vi "Main Page.vi"(8 "error in (no error)":errorcluster, 11 "Node Ptr":T2 format="%.0x") -> (0 "error out":errorcluster)   [LabVIEW 2015, in "SLSC-12201 DIO System Explorer.lvlib"]
uses:
  SLSC-12201 DIO System Explorer.lvlib
  <vilib>/NI Veristand/Custom Device API/Custom Device Item Ref.ctl
  Direction Control.ctl
  Shared/Constants.vi
  <vilib>/NI Veristand/Custom Device Tools/Custom Device Utility Library/NI VeriStand - Search for All Items by Name.vi
  <vilib>/NI Veristand/Custom Device API/Get Item Property (Boolean).vi
  <vilib>/NI Veristand/Custom Device Tools/Custom Device Utility Library/NI VeriStand - Search for Item by Name.vi
  <vilib>/NI Veristand/Custom Device API/Get Item Property (I32).vi
  <vilib>/NI Veristand/Custom Device API/Get Item Property (Variant).vi
  <vilib>/NI Veristand/Custom Device API/Set Item Property (Variant).vi
  SLSC Pinout Window.vi
  SLSC Diagram Window.vi
  <vilib>/NI Veristand/Custom Device API/Set Item Property (Boolean).vi
  <vilib>/NI Veristand/Custom Device API/Set Item Property (String).vi
  <vilib>/NI Veristand/Custom Device API/Custom Device API.lvlib
  Shared/SLSC-12201 DIO Shared.lvlib
  <vilib>/NI Veristand/Custom Device Tools/Custom Device Utility Library/Custom Device Utility Library.lvlib
panel:
  in  "Loop rate":u32
  in  "rev A":bool
  in  "SHDocVw.IWebBrowser2":refnum<k7>(container)
  out "Version":string
  in  "Direction":T1 items=["Input", "Output Source", "Output Sink", "Output Push-Pull"]
  in  "Apply":bool
  in  "Enable":bool
  in  "Disable":bool
  in  "Tab Control":enum32{"Bank 0", "Bank 1"}(tab)
  in  "Input Threshold 5V Bank 0":dbl caption="Input Threshold"
  in  "Bank0 Select Vsup":u16(ring) caption="Voltage Supply" items=["Off", "Vsup_0", "Vsup_1"]
  in  "Pullup Resistor Bank 0":bool
  in  "Input Threshold 33V Bank 0":dbl caption="Input Threshold"
  in  "Enable 5V Range Bank 0":bool
  in  "Input Threshold 5V Bank 1":dbl caption="Input Threshold"
  in  "Bank1 Select Vsup":u16(ring) caption="Voltage Supply" items=["Off", "Vsup_0", "Vsup_1"]
  in  "Enable 5V Range Bank 1":bool
  in  "Pullup Resistor Bank 1":bool
  in  "Input Threshold 33V Bank 1":dbl caption="Input Threshold"
  in  "Tree":string[](tree)
  in  "Make Static Only":bool
  in  "Title":cluster{"Section Name":string}={"Section Name"="Custom Device Properties"}
  out "Module Number":i32
  in  "Header":cluster{"Section Name":string}={"Section Name"="Custom Device Item Settings"}
  in  "Description":string
  in  "Name":string
  # "ms"
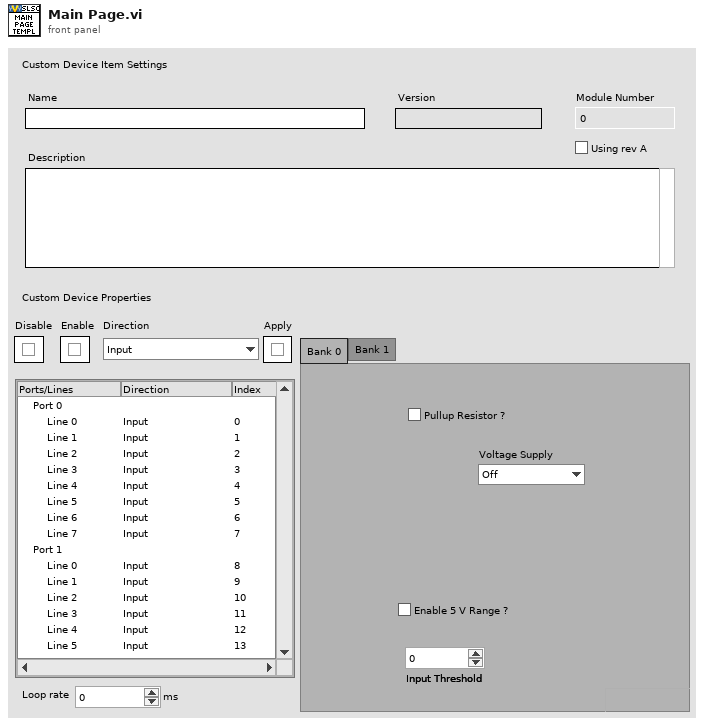
[diagram p1: front panel]
types:
  T1 = typedef "SLSC-12201 DIO System Explorer.lvlib/Direction Control.ctl" = u16
  T2 = typedef "Custom Device API.lvlib/Custom Device Item Ref.ctl" = u64
  T3 = enum8{"Enabled", "Disabled", "Disabled and Grayed Out"}
  T4 = typedef "Custom Device API.lvlib/Custom Device Channel.ctl" = cluster{"Type":T5, "Units":string, "Default Value":dbl, "Faultable":bool, "Scalable":bool}
  T5 = typedef "Custom Device API.lvlib/Custom Device Channel Type.ctl" = enum16{"Input", "Output"}
  T6 = cluster{"Channel Name":string, "SLSC Name":string, "Channel":T4, "Enum Names":string[], "Enum Values":i32[]}[]
  T7 = typedef "SLSC-12201 DIO System Explorer.lvlib/SLSC Channel Information.ctl" = cluster{"Channel Name":string, "SLSC Name":string, "Configuration":T4, "Enum Names":string[], "Enum Values":i32[]}
  T8 = typedef "Custom Device API.lvlib/Custom Device Item Info.ctl" = cluster{"Name":string, "Is Channel":bool, "GUID":string, "Is Waveform":bool}
  T9 = typedef "Custom Device API.lvlib/Custom Device Commands.ctl" = enum16{"Default", "Item renamed", "Shutdown", "Dynamic button pressed"}
  T10 = typedef "LVPoint32TypeDef.ctl" = cluster{"Horizontal":i32, "Vertical":i32}
  T11 = cluster{"Channel Name":string, "SLSC Name":string, "Channel":T4}[]
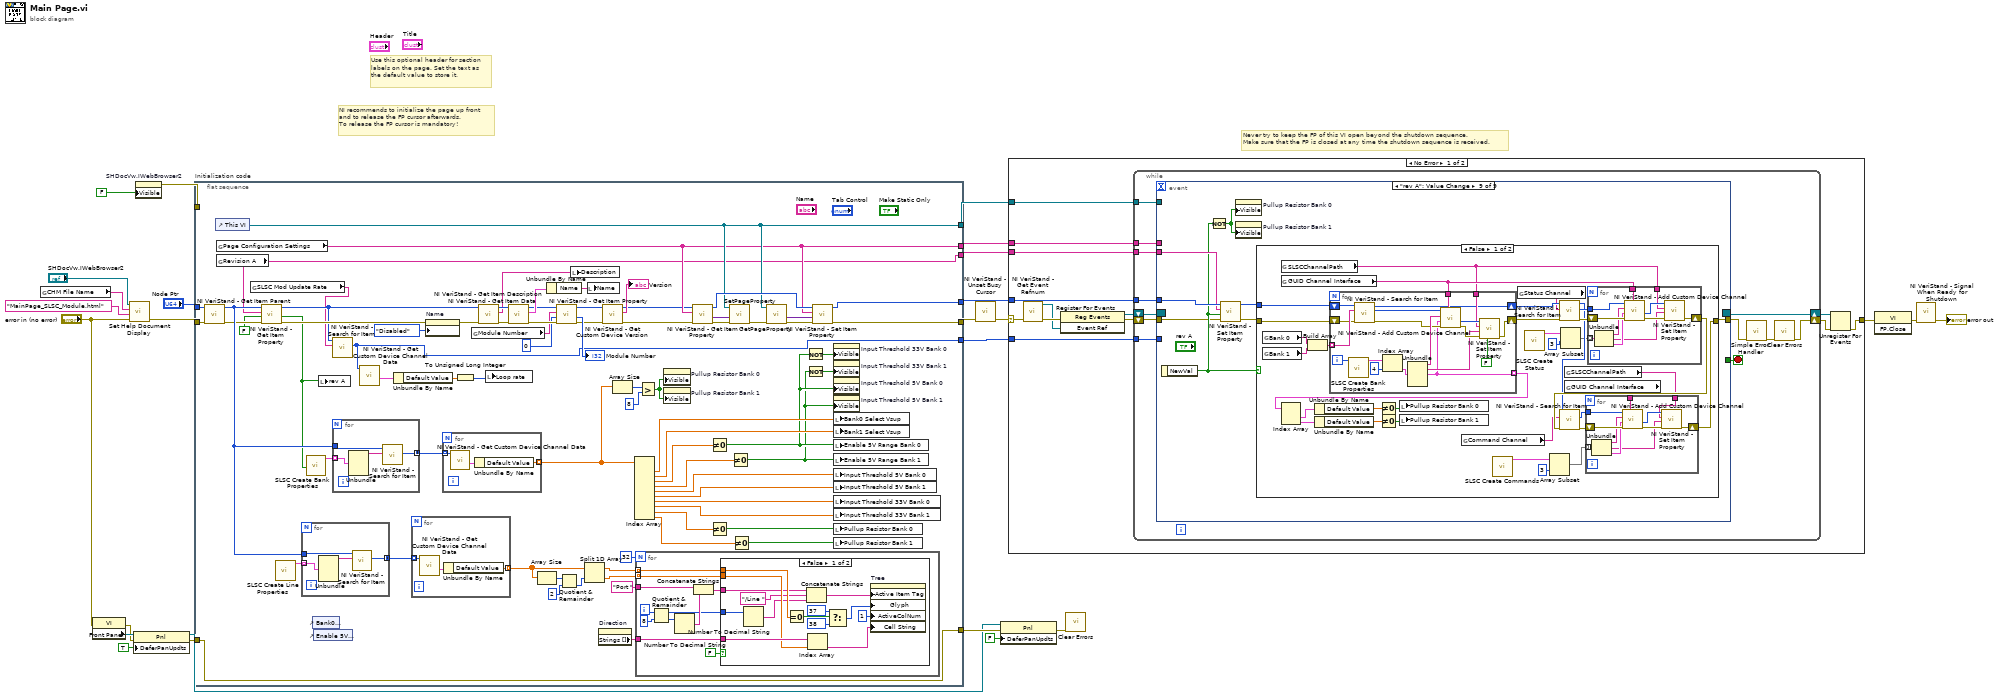
[diagram p0: block diagram]
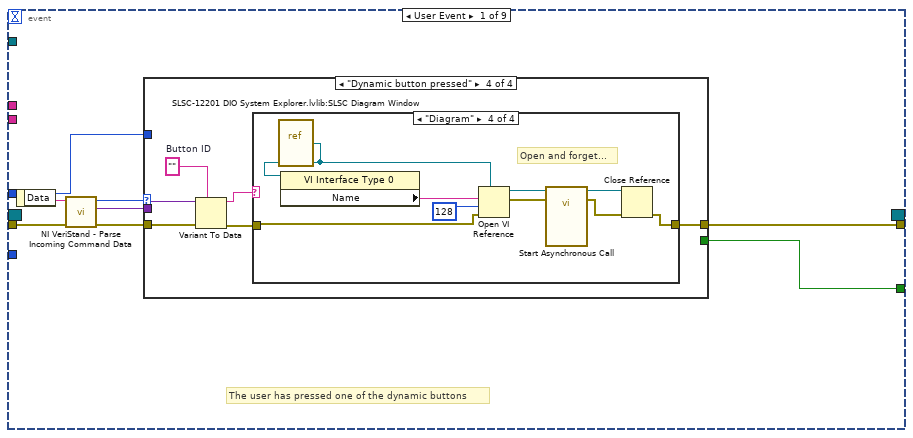
[diagram p2: hidden frame]
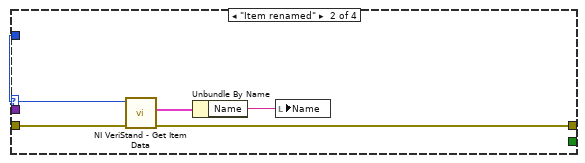
[diagram p4: hidden frame]
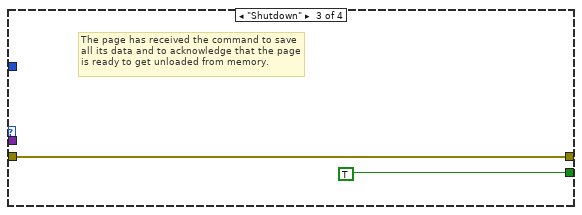
[diagram p5: hidden frame]
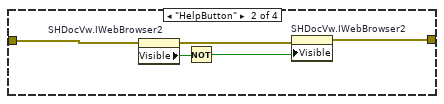
[diagram p7: hidden frame]
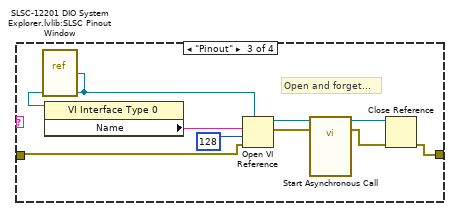
[diagram p8: hidden frame]
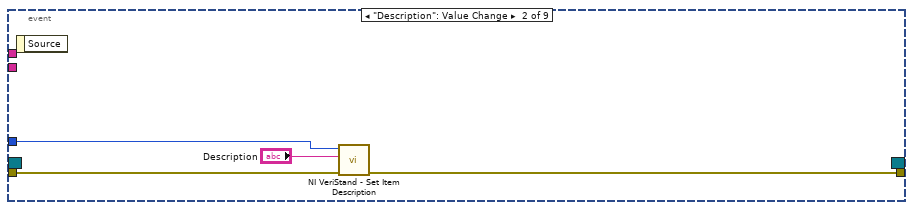
[diagram p9: hidden frame]
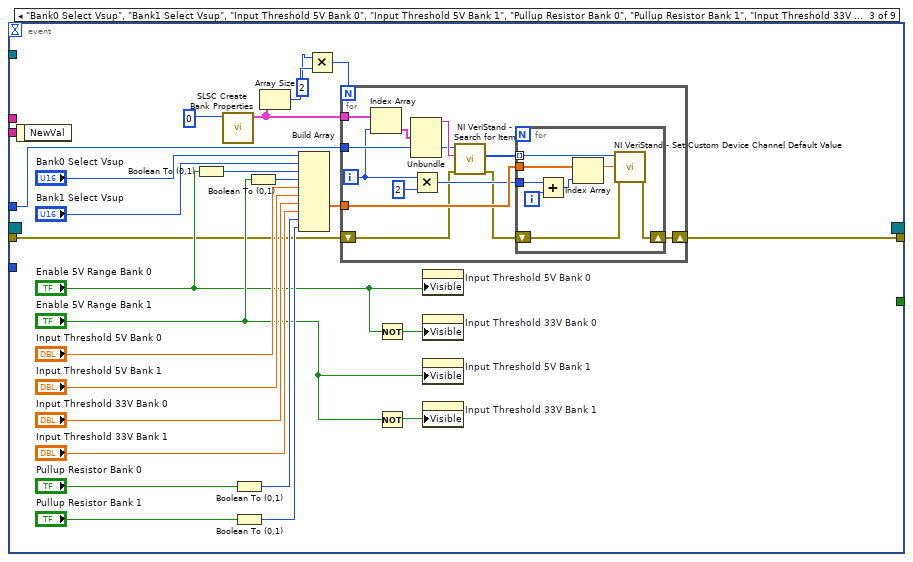
[diagram p10: hidden frame]
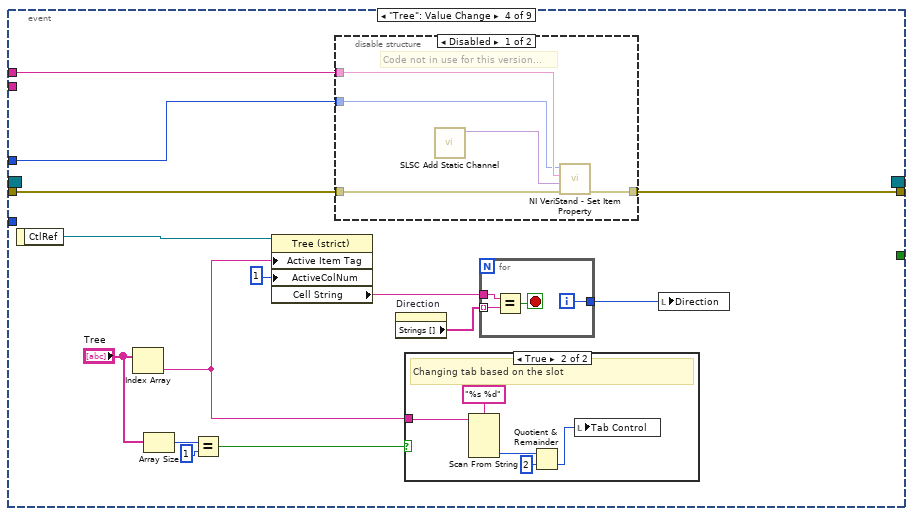
[diagram p11: hidden frame]
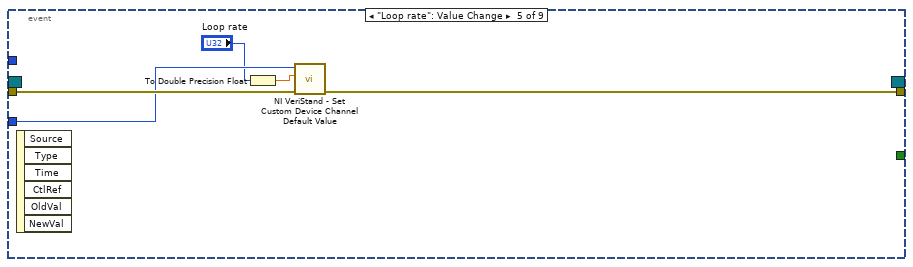
[diagram p14: hidden frame]
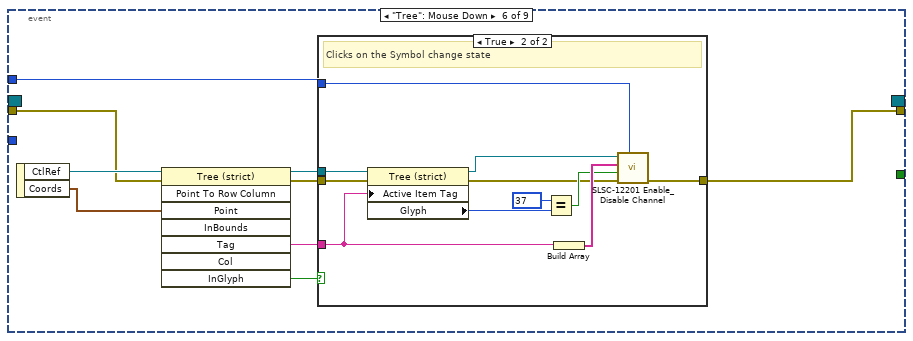
[diagram p15: hidden frame]
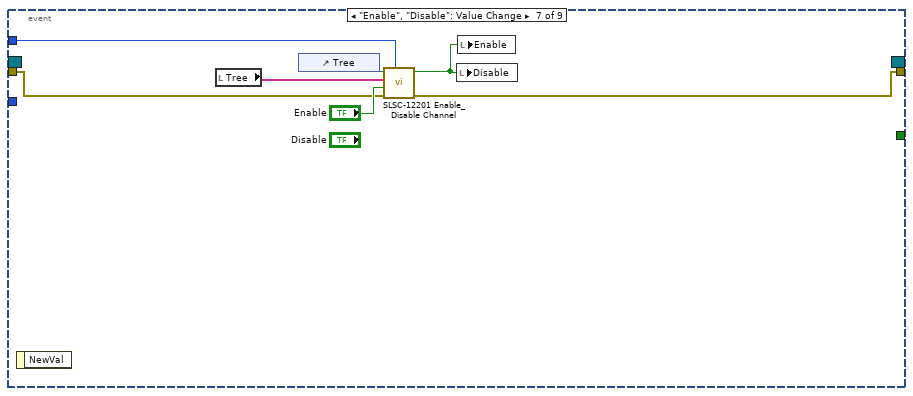
[diagram p17: hidden frame]
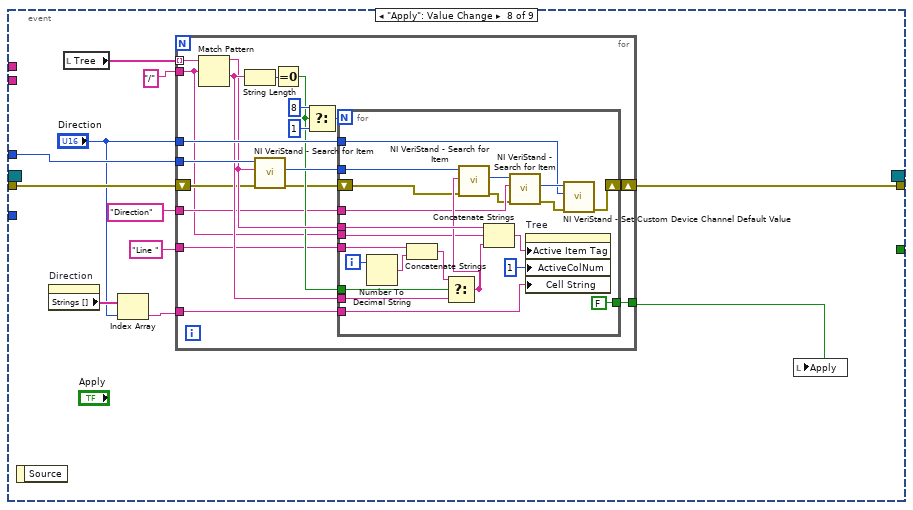
[diagram p18: hidden frame]
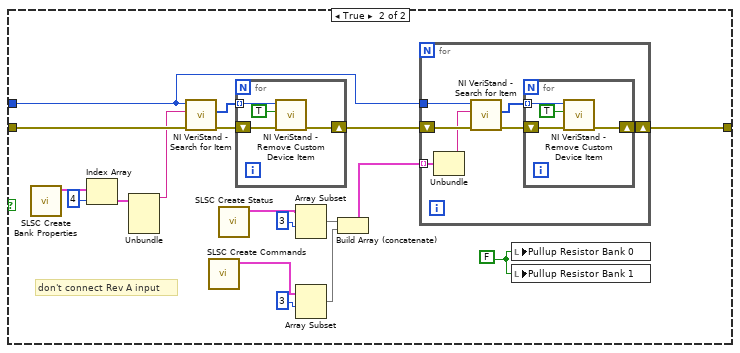
[diagram p19: hidden frame]
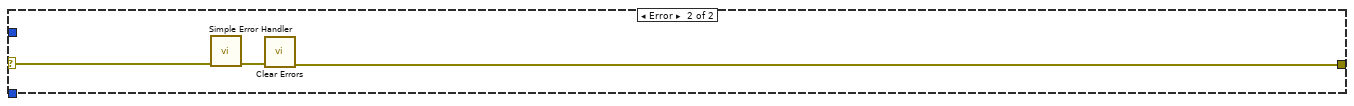
[diagram p20: hidden frame]
diagram:
  # "Never try to keep the FP of this VI open beyond the shutdown sequence.\nMake sure that the FP is closed at any time the shutdown sequence is received."
  # "Use this optional header for section labels on the page. Set the text as the default value to store it."
  # "NI recommends to initialize the page up front\nand to release the FP cursor afterwards.\nTo release the FP cursor is mandatory!"
  n1 = global read "Constants.vi" "CHM File Name"() -> (w13:string)
  n2 = property class="VI"(error in="error in (no error)") -> (error out=w8:errorcluster, "Front Panel"=w10:refnum<vi>)  [unwired: 1 in, 1 out]
  n3 = call "Set Help Document Display.vi"("error in (no error)"="error in (no error)", "HTML File"="MainPage_SLSC_Module.html", "Main CHM File"=w13, "SHDocVw.IWebBrowser2"="SHDocVw.IWebBrowser2") -> ("error out"=w14:errorcluster)  [unwired: 7 in]
  n4 = property class="Pnl"(reference=w10, error in=w8, "DeferPanUpdts"=TRUE ("Defer Panel Updates")) -> (reference out=w2:refnum<vi>, error out=w6:errorcluster)
  n5 = property on="SHDocVw.IWebBrowser2" class="AXCont"("Visible"=FALSE) -> (error out=w17:errorcluster)  [unwired: 2 in, 1 out]
  n6 = flat-sequence "Initialization code" {
    tunnel: w14 -> [w78]
    tunnel: "Node Ptr" -> [w79]
    tunnel: [w85] -> w22
    tunnel: [w82] -> w20
    tunnel: [w81] -> w19
    tunnel: [w80] -> w18
    tunnel: w17 -> [_]
    tunnel: [w35] -> w16
    tunnel: w6 -> [w33]
    tunnel: [w33] -> w4
    tunnel: [w27] -> w1
    frame #0 {
      n7 = call <vilib>:"NI VeriStand - Get Item Parent.vi"("error in (no error)"=w78, "Item Ref in"=w79) -> ("error out"=w38:errorcluster, "Item Ref out"=w39:T2)  [unwired: 6 in, 2 out]
      n8 = control-ref of="This VI"() -> (w81:refnum<vi>)
      n9 = global read "Constants.vi" "Page Configuration Settings"() -> (w80:string)
      n10 = global read "Constants.vi" "Revision A"() -> (w35:string)
      n11 = global read "Constants.vi" "SLSC Mod Update Rate"() -> (w28:string)
      n12 = call-poly <vilib>:"NI VeriStand - Get Item Property.vi"("error in (no error)"=w38, "Default Value"=FALSE, "Property Name"=w35, "Item Ref in"=w39) -> ("error out"=w37:errorcluster, "Value"=w34:bool, "Item Ref out"=w32:T2)  [unwired: 4 in, 1 out]
      n13 = call "SLSC Create Line Properties.vi"() -> ("Outgoing configuration"=w67:T6)  [unwired: 11 in]
      n14 = for {
        tunnel: w39 -> [w133]
        tunnel: w67 -> [w132] mode=indexing
        tunnel: [w131] -> w66 mode=concatenating
        n15 = Unbundle(w132) -> ("Channel Name"=w130:string)  [unwired: 4 out]
        n16 = call-poly <vilib>:"NI VeriStand - Search for Item.vi"("Item Name"=w130, "Section Ref in"=w133) -> ("Item Refs"=w131:T2[])  [unwired: 6 in, 3 out]
      }
      n17 = call "SLSC Create Bank Properties.vi"("RevA?"=w34) -> ("Outgoing configuration"=w74:T7[])  [unwired: 9 in, 1 out]
      n18 = control-ref of="Bank0 Select Vsup"() -> ()  [unwired: 1 out]
      n19 = control-ref of="Enable 5V Range Bank 0"() -> ()  [unwired: 1 out]
      n20 = local write "rev A"(w34) -> ()
      n21 = call-poly <vilib>:"NI VeriStand - Search for Item.vi"("Item Name"=w28, "Section Ref in"=w32) -> ("Item Ref"=w27:T2)  [unwired: 6 in, 3 out]
      n22 = for {
        tunnel: w39 -> [w137]
        tunnel: w74 -> [w135] mode=indexing
        tunnel: [w134] -> w73 mode=concatenating
        n23 = Unbundle(w135) -> ("Channel Name"=w136:string)  [unwired: 4 out]
        n24 = call-poly <vilib>:"NI VeriStand - Search for Item.vi"("Item Name"=w136, "Section Ref in"=w137) -> ("Item Refs"=w134:T2[])  [unwired: 6 in, 3 out]
      }
      n25 = call <vilib>:"NI VeriStand - Get Custom Device Channel Data.vi"("Channel Ref in"=w27) -> ("Channel"=w31:T4)  [unwired: 5 in, 5 out]
      n26 = Unbundle By Name(w31) -> ("Default Value"=w30:dbl)
      n27 = for {
        tunnel: [w129] -> w60 mode=indexing
        tunnel: w66 -> [w128] mode=indexing
        n28 = call <vilib>:"NI VeriStand - Get Custom Device Channel Data.vi"("Channel Ref in"=w128) -> ("Channel"=w127:T4)  [unwired: 5 in, 5 out]
        n29 = Unbundle By Name(w127) -> ("Default Value"=w129:dbl)
      }
      n30 = property on="Name" class="Str"(error in=w37, "DisabledEnum"=T3."Disabled" ("Disabled")) -> (error out=w95:errorcluster)  [unwired: 1 in, 1 out]
      n31 = for {
        tunnel: [w140] -> w52 mode=indexing
        tunnel: w73 -> [w139] mode=indexing
        n32 = call <vilib>:"NI VeriStand - Get Custom Device Channel Data.vi"("Channel Ref in"=w139) -> ("Channel"=w138:T4)  [unwired: 5 in, 5 out]
        n33 = Unbundle By Name(w138) -> ("Default Value"=w140:dbl)
      }
      n34 = To Unsigned Long Integer(number=w30) -> (unsigned 32bit integer=w29:u32)
      n35 = global read "Constants.vi" "Module Number"() -> (w92:string)
      n36 = call <vilib>:"NI VeriStand - Get Item Description.vi"("error in (no error)"=w95, "Item Ref in"=w32) -> ("error out"=w99:errorcluster, "Description"=w100:string, "Item Ref out"=w101:T2)  [unwired: 7 out]
      n37 = local write "Loop rate"(w29) -> ()
      n38 = call <vilib>:"NI VeriStand - Get Item Data.vi"("error in (no error)"=w99, "Item Ref in"=w101) -> ("error out"=w93:errorcluster, "Item Info"=w98:T8, "Item Ref out"=w91:T2)  [unwired: 7 out]
      n39 = Array Size(array=w60) -> (size(s)=w59:i32)
      n40 = Unbundle By Name(w98) -> ("Name"=w97:string)
      n41 = call-poly <vilib>:"NI VeriStand - Get Item Property.vi"("error in (no error)"=w93, "Default Value"=0, "Property Name"=w92, "Item Ref in"=w91) -> ("error out"=w43:errorcluster, "Value"=→"Module Number":i32, "Item Ref out"=w41:T2)  [unwired: 4 in, 1 out]
      n42 = Quotient & Remainder(x=w59, y=2) -> (floor(x/y)=w57:i32)  [unwired: 1 out]
      n43 = local write "Description"(w100) -> ()
      n44 = Split 1D Array(array=w60, index=w57) -> (first subarray=w65:dbl[], second subarray=w64:dbl[])
      n45 = local write "Name"(w97) -> ()
      n46 = property on="Direction" class="Ring (strict)"() -> ("Strings []"=w63:string[])  [unwired: 2 in, 2 out]
      n47 = call <vilib>:"NI VeriStand - Get Custom Device Version.vi"("error in (no error)"=w43, "Device Ref in"=w41) -> ("error out"=w42:errorcluster, "Value"=→"Version":string, "Device Ref out"=w40:T2)  [unwired: 7 in]
      n48 = Array Size(array=w52) -> (size(s)=w51:i32)
      n49 = Index Array(array=w52) -> (element #1=w77:dbl, element #2=w72:dbl, element #3=w71:dbl, element #4=w70:dbl, element #5=w56:dbl, element #6=w55:dbl, element #7=w54:dbl, element #8=w53:dbl, element #9=w69:dbl, element #10=w68:dbl)  [unwired: 10 in]
      n50 = for {
        N: 32 -> [_]
        tunnel: w65 -> [w112] mode=indexing
        tunnel: w64 -> [w110] mode=indexing
        tunnel: w63 -> [w111]
        tunnel: "Port " ("y") -> [w106]
        i -> [w109]
        n51 = Quotient & Remainder(x=w109, y=8) -> (x-y*floor(x/y)=w103:i32, floor(x/y)=w107:i32)
        n52 = Number To Decimal String(number=w107) -> (decimal integer string=w105:string)  [unwired: 1 in]
        n53 = Concatenate Strings(w106, w105) -> (w104:string)
        n54 = case shown="False" FALSE {
          tunnel: w112 -> [w122 _]
          tunnel: w111 -> [w120 _]
          tunnel: w110 -> [w119 _]
          tunnel: w104 -> [w115 _]
          tunnel: w103 -> [w113 _]
          frame False {
            n55 = Number To Decimal String(number=w113) -> (decimal integer string=w116:string)  [unwired: 1 in]
            n56 = Equal To 0?(x=w122) -> (x = 0?=w124:bool)
            n57 = Concatenate Strings(w115, "/Line " ("string"), w116) -> (w114:string)
            n58 = Index Array(array=w120, index=w119) -> (element=w118:string)
            n59 = Select(t=37, s=w124, f=38) -> (s? t:f=w123:i32)
            n60 = property on="Tree" class="Tree (strict)"("Active Item Tag"=w114, "Glyph"=w123, "ActiveColNum"=1 ("Active Cell:Active Column Number"), "Cell String"=w118) -> ()  [unwired: 2 in, 2 out]
          }
          frame True {
          }
        }
      }
      n61 = Greater?(x=w51, y=8) -> (0:w45:bool)
      n62 = property on="Pullup Resistor Bank 0" class="Bool (strict)"("Visible"=w45) -> ()  [unwired: 2 in, 2 out]
      n63 = property on="Pullup Resistor Bank 1" class="Bool (strict)"("Visible"=w45) -> ()  [unwired: 2 in, 2 out]
      n64 = call-poly <vilib>:"NI VeriStand - Get Item Property.vi"("error in (no error)"=w42, "Property Name"=w80, "Item Ref in"=w40) -> ("error out"=w89:errorcluster, "Value"=w88:variant, "Item Ref out"=w84:T2)  [unwired: 5 in, 1 out]
      n65 = Not Equal To 0?(x=w71) -> (x != 0?=w47:bool)
      n66 = Not Equal To 0?(x=w69) -> (x != 0?=w76:bool)
      n67 = call "SetPageProperty.vi"("error in"=w89, "variant"=w88, "This VI"=w81) -> ("error out"=w87:errorcluster)  [unwired: 8 in]
      n68 = Not Equal To 0?(x=w70) -> (x != 0?=w46:bool)
      n69 = Not Equal To 0?(x=w68) -> (x != 0?=w75:bool)
      n70 = call "GetPageProperty.vi"("error in (no error)"=w87, "This VI"=w81) -> ("error out"=w86:errorcluster, "Settings"=w83:variant)  [unwired: 8 in]
      n71 = Not(x=w47) -> (.not. x?=w49:bool)
      n72 = Not(x=w46) -> (.not. x?=w48:bool)
      n73 = call-poly <vilib>:"NI VeriStand - Set Item Property.vi"("error in (no error)"=w86, "Value"=w83, "Property Name"=w80, "Item Ref in"=w84) -> ("error out"=w85:errorcluster, "Item Ref out"=w82:T2)  [unwired: 5 in, 1 out]
      n74 = property on="Input Threshold 33V Bank 0" class="DigNum (strict)"("Visible"=w49) -> ()  [unwired: 2 in, 2 out]
      n75 = property on="Input Threshold 33V Bank 1" class="DigNum (strict)"("Visible"=w48) -> ()  [unwired: 2 in, 2 out]
      n76 = property on="Input Threshold 5V Bank 0" class="DigNum (strict)"("Visible"=w47) -> ()  [unwired: 2 in, 2 out]
      n77 = property on="Input Threshold 5V Bank 1" class="DigNum (strict)"("Visible"=w46) -> ()  [unwired: 2 in, 2 out]
      n78 = local write "Bank0 Select Vsup"(w77) -> ()
      n79 = local write "Bank1 Select Vsup"(w72) -> ()
      n80 = local write "Enable 5V Range Bank 0"(w47) -> ()
      n81 = local write "Enable 5V Range Bank 1"(w46) -> ()
      n82 = local write "Input Threshold 5V Bank 0"(w56) -> ()
      n83 = local write "Input Threshold 5V Bank 1"(w55) -> ()
      n84 = local write "Input Threshold 33V Bank 0"(w54) -> ()
      n85 = local write "Input Threshold 33V Bank 1"(w53) -> ()
      n86 = local write "Pullup Resistor Bank 0"(w76) -> ()
      n87 = local write "Pullup Resistor Bank 1"(w75) -> ()
    }
  }
  n88 = call <vilib>:"NI VeriStand - Unset Busy Cursor.vi"("error in (no error)"=w22) -> ("error out"=w21:errorcluster)  [unwired: 10 out]
  n89 = property class="Pnl"(reference=w2, error in=w4, "DeferPanUpdts"=FALSE ("Defer Panel Updates")) -> (error out=w3:errorcluster)  [unwired: 1 out]
  n90 = case shown="No Error" w21 {
    selector: w21 -> [w145 w492]
    tunnel: [w150 w490] -> w26
    tunnel: w20 -> [w146 _]
    tunnel: w19 -> [w144 _]
    tunnel: w18 -> [w143 _]
    tunnel: w16 -> [w142 _]
    tunnel: w1 -> [w141 _]
    frame No Error {
      n91 = call <vilib>:"NI VeriStand - Get Event Refnum.vi"("error in (no error)"=w145) -> ("error out"=w153:errorcluster, "Event Ref"=w149:refnum<user-event>)  [unwired: 9 out]
      n92 = register-events(error in=w153, w149) -> (reference out=w147:refnum<event-registration>, error out=w148:errorcluster)  [unwired: 1 in]
      n93 = while {
        tunnel: w146 -> [w161]
        shift-right: [w158] -> w151
        shift-left: w148 -> [w164]
        shift-right: [w165] -> w152
        shift-left: w147 -> [w163]
        tunnel: w144 -> [w157]
        tunnel: w143 -> [w156]
        tunnel: w142 -> [w155]
        tunnel: w141 -> [w154]
        stop <- w162 stop-if-true
        n94 = event shown="[8] \"rev A\": Value Change" {
          selector: w163 -> [_ _ _ _ _ _ _ _ _]
          dyn-events: [_ _ _ _ _ _ _ _ _] -> w165
          timeout: _ -> [_ _ _ _ _ _ _ _ _]
          tunnel: w164 -> [w173 w214 w217 w273 w293 w301 w318 w327 w376]
          tunnel: [w169 _ _ _ _ _ _ _ _] -> w162
          tunnel: [w168 w213 w216 w274 w292 w297 w317 w326 w382] -> w160
          tunnel: w161 -> [w167 w215 w239 w271 _ w298 w321 w332 w380]
          tunnel: w157 -> [_ _ _ _ _ _ _ _ _]
          tunnel: w156 -> [_ _ _ w272 _ _ _ _ _]
          tunnel: w155 -> [_ _ _ _ _ _ _ _ w378]
          tunnel: w154 -> [_ _ _ _ w291 _ _ _ _]
          event User Event {
            # "The user has pressed one of the dynamic buttons"
            n95 = event-data() -> ("Data"=w172:string)  [unwired: 1 out]
            n96 = call <vilib>:"NI VeriStand - Parse Incoming Command Data.vi"("error in (no error)"=w173, "Incoming data"=w172) -> ("error out"=w171:errorcluster, "Outgoing data"=w166:variant, "Action"=w170:T9)  [unwired: 7 out]
            n97 = case shown="\"Dynamic button pressed\"" w170 {
              tunnel: w171 -> [w174 w179 w180 w187]
              tunnel: [_ _ TRUE _] -> w169
              tunnel: [w174 w176 w180 w182] -> w168
              tunnel: w167 -> [_ w178 _ _]
              tunnel: w166 -> [_ _ _ w186]
              frame "Default", Default {
              }
              frame "Item renamed" {
                n98 = call <vilib>:"NI VeriStand - Get Item Data.vi"("error in (no error)"=w179, "Item Ref in"=w178) -> ("error out"=w176:errorcluster, "Item Info"=w177:T8)  [unwired: 8 out]
                n99 = Unbundle By Name(w177) -> ("Name"=w175:string)
                n100 = local write "Name"(w175) -> ()
              }
              frame "Shutdown" {
                # "The page has received the command to save all its data and to acknowledge that the page is ready to get unloaded from memory."
              }
              frame "Dynamic button pressed" {
                w185 = ""  # Button ID
                n101 = Variant To Data(error in=w187, type=w185, Variant=w186) -> (data=w184:string, error out=w183:errorcluster)
                n102 = case shown="\"Diagram\"" w184 {
                  tunnel: w183 -> [w188 w191 w195 w204]
                  tunnel: [w188 w189 w196 w205] -> w182
                  frame Default {
                  }
                  frame "HelpButton" {
                    n103 = property on="SHDocVw.IWebBrowser2" class="AXCont"(error in=w191) -> (error out=w190:errorcluster, "Visible"=w193:bool)  [unwired: 1 in, 1 out]
                    n104 = Not(x=w193) -> (.not. x?=w192:bool)
                    n105 = property on="SHDocVw.IWebBrowser2" class="AXCont"(error in=w190, "Visible"=w192) -> (error out=w189:errorcluster)  [unwired: 1 in, 1 out]
                  }
                  frame "Pinout" {
                    # "Open and forget..."
                    n106 = vi-ref "SLSC-12201 DIO System Explorer.lvlib:SLSC Pinout Window.vi"() -> (w194:refnum<vi>)
                    n107 = property class="VI Interface Type 0"(reference=w194) -> ("Name"=w202:string)  [unwired: 1 in, 2 out]
                    n108 = Open VI Reference(type specifier VI Refnum (for type only)=w194, vi path=w202, options=128, error in (no error)=w195) -> (vi reference=w198:refnum<vi>, error out=w200:errorcluster)  [unwired: 2 in]
                    n109 = call-by-ref "Start Asynchronous Call"(reference=w198, error in=w200) -> (reference out=w199:refnum<vi>, error out=w201:errorcluster)  [unwired: 12 in]
                    n110 = Close Reference(reference=w199, error in (no error)=w201) -> (error out=w196:errorcluster)
                  }
                  frame "Diagram" {
                    # "Open and forget..."
                    n111 = vi-ref "SLSC-12201 DIO System Explorer.lvlib:SLSC Diagram Window.vi"() -> (w203:refnum<vi>)
                    n112 = property class="VI Interface Type 0"(reference=w203) -> ("Name"=w211:string)  [unwired: 1 in, 2 out]
                    n113 = Open VI Reference(type specifier VI Refnum (for type only)=w203, vi path=w211, options=128, error in (no error)=w204) -> (vi reference=w207:refnum<vi>, error out=w209:errorcluster)  [unwired: 2 in]
                    n114 = call-by-ref "Start Asynchronous Call"(reference=w207, error in=w209) -> (reference out=w208:refnum<vi>, error out=w210:errorcluster)  [unwired: 12 in]
                    n115 = Close Reference(reference=w208, error in (no error)=w210) -> (error out=w205:errorcluster)
                  }
                }
              }
            }
          }
          event "Description": Value Change {
            n116 = event-data() -> ()  [unwired: 2 out]
            n117 = call <vilib>:"NI VeriStand - Set Item Description.vi"("error in (no error)"=w214, "Description"="Description", "Item Ref in"=w215) -> ("error out"=w213:errorcluster)  [unwired: 8 out]
          }
          event "Bank0 Select Vsup", "Bank1 Select Vsup", "Input Threshold 5V Bank 0", "Input Threshold 5V Bank 1", "Pullup Resistor Bank 0", "Pullup Resistor Bank 1", "Input Threshold 33V Bank 0", "Input Threshold 33V Bank 1", "Enable 5V Range Bank 1", "Enable 5V Range Bank 0": Value Change {
            n118 = event-data() -> ()  [unwired: 2 out]
            n119 = Boolean To (0,1)(Boolean="Enable 5V Range Bank 0") -> (0, 1=w235:i16)
            n120 = call "SLSC Create Bank Properties.vi"("Bank Number"=0) -> ("Outgoing configuration"=w225:T7[])  [unwired: 9 in, 1 out]
            n121 = Boolean To (0,1)(Boolean="Pullup Resistor Bank 0") -> (0, 1=w227:i16)
            n122 = Boolean To (0,1)(Boolean="Pullup Resistor Bank 1") -> (0, 1=w226:i16)
            n123 = Boolean To (0,1)(Boolean="Enable 5V Range Bank 1") -> (0, 1=w234:i16)
            n124 = Array Size(array=w225) -> (size(s)=w223:i32)
            n125 = Build Array("Bank0 Select Vsup", "Bank1 Select Vsup", w235, w234, "Input Threshold 5V Bank 0", "Input Threshold 5V Bank 1", "Input Threshold 33V Bank 0", "Input Threshold 33V Bank 1", w227, w226) -> (w236:dbl[])
            n126 = Multiply(x=2 ("y"), y=w223) -> (x*y=w224:i32)
            n127 = for {
              N: w224 -> [_]
              tunnel: w239 -> [w251]
              tunnel: w236 -> [w249]
              tunnel: w225 -> [w248]
              shift-right: [w241] -> w216
              shift-left: w217 -> [w243]
              i -> [w245]
              n128 = Index Array(array=w248, index=w245) -> (element=w247:T7)
              n129 = Unbundle(w247) -> ("Channel Name"=w252:string)  [unwired: 4 out]
              n130 = Multiply(x=w245, y=2) -> (x*y=w244:i32)
              n131 = call-poly <vilib>:"NI VeriStand - Search for Item.vi"("error in"=w243, "Item Name"=w252, "Section Ref in"=w251) -> ("error out"=w242:errorcluster, "Item Refs"=w250:T2[])  [unwired: 5 in, 2 out]
              n132 = for {
                tunnel: w249 -> [w260]
                tunnel: w250 -> [w259] mode=indexing
                tunnel: w244 -> [w255]
                shift-right: [w253] -> w241
                shift-left: w242 -> [w254]
                i -> [w257]
                n133 = Add(x=w255, y=w257) -> (x+y=w256:i32)
                n134 = Index Array(array=w260, index=w256) -> (element=w258:dbl)
                n135 = call <vilib>:"NI VeriStand - Set Custom Device Channel Default Value.vi"("error in (no error)"=w254, "Default Value"=w258, "Channel Ref in"=w259) -> ("error out"=w253:errorcluster)  [unwired: 7 in, 1 out]
              }
            }
            n136 = Not(x="Enable 5V Range Bank 0") -> (.not. x?=w221:bool)
            n137 = Not(x="Enable 5V Range Bank 1") -> (.not. x?=w220:bool)
            n138 = property on="Input Threshold 5V Bank 0" class="DigNum (strict)"("Visible"="Enable 5V Range Bank 0") -> ()  [unwired: 2 in, 2 out]
            n139 = property on="Input Threshold 33V Bank 0" class="DigNum (strict)"("Visible"=w221) -> ()  [unwired: 2 in, 2 out]
            n140 = property on="Input Threshold 5V Bank 1" class="DigNum (strict)"("Visible"="Enable 5V Range Bank 1") -> ()  [unwired: 2 in, 2 out]
            n141 = property on="Input Threshold 33V Bank 1" class="DigNum (strict)"("Visible"=w220) -> ()  [unwired: 2 in, 2 out]
          }
          event "Tree": Value Change {
            n142 = event-data() -> ("CtlRef"=w270:refnum<vi>)  [unwired: 1 out]
            n143 = Index Array(array="Tree") -> (element=w261:string)  [unwired: 1 in]
            n144 = Array Size(array="Tree") -> (size(s)=w264:i32)
            n145 = Equal?(x=w264, y=1) -> (x = y?=w262:bool)
            n146 = property on="Property Node" class="Tree (strict)"(reference=w270, "Active Item Tag"=w261, "ActiveColNum"=1 ("Active Cell:Active Column Number")) -> ("Cell String"=w267:string)  [unwired: 1 in, 2 out]
            n147 = disable-structure shown="Disabled" {
              disable-tunnel: [w288 w289] -> w274
              disable-tunnel: w273 -> [w287 w289]
              disable-tunnel: w272 -> [w285 _]
              disable-tunnel: w271 -> [w284 _]
              frame Disabled {
                # "Code not in use for this version..."
                n148 = call "SLSC Add Static Channel.vi"() -> ("variant out"=w286:variant)  [unwired: 10 in, 1 out]
                n149 = call-poly <vilib>:"NI VeriStand - Set Item Property.vi"("error in (no error)"=w287, "Value"=w286, "Property Name"=w285, "Item Ref in"=w284) -> ("error out"=w288:errorcluster)  [unwired: 5 in, 2 out]
              }
              frame Enabled {
              }
            }
            n150 = property on="Direction" class="Ring (strict)"() -> ("Strings []"=w268:string[])  [unwired: 2 in, 2 out]
            n151 = case shown="True" w262 {
              tunnel: w261 -> [_ w278]
              frame False {
              }
              frame True {
                # "Changing tab based on the slot"
                n152 = Scan From String(format string="%s %d", input string=w278) -> (output 2=w277:i32)  [unwired: 5 in, 3 out]
                n153 = Quotient & Remainder(x=w277, y=2) -> (floor(x/y)=w275:i32)  [unwired: 1 out]
                n154 = local write "Tab Control"(w275) -> ()
              }
            }
            n155 = for {
              tunnel: w268 -> [w283] mode=indexing
              tunnel: w267 -> [w282]
              tunnel: [w280] -> w266
              i -> [w280]
              stop <- w281 stop-if-true
              n156 = Equal?(x=w282, y=w283) -> (x = y?=w281:bool)
            }
            n157 = local write "Direction"(w266) -> ()
          }
          event "Loop rate": Value Change {
            n158 = event-data() -> ()  [unwired: 7 out]
            n159 = To Double Precision Float(number="Loop rate") -> (double precision float=w294:dbl)
            n160 = call <vilib>:"NI VeriStand - Set Custom Device Channel Default Value.vi"("error in (no error)"=w293, "Default Value"=w294, "Channel Ref in"=w291) -> ("error out"=w292:errorcluster)  [unwired: 7 in, 1 out]
          }
          event "Tree": Mouse Down {
            n161 = event-data() -> ("CtlRef"=w303:refnum<vi>, "Coords"=w302:T10)  [unwired: 1 out]
            n162 = invoke class="Tree (strict)" method="Point To Row Column"(reference=w303, error in=w301, "Point"=w302) -> (reference out=w296:refnum<vi>, error out=w295:errorcluster, "Tag"=w299:string, "InGlyph"=w300:bool)  [unwired: 5 in, 4 out]
            n163 = case shown="True" w300 {
              tunnel: w299 -> [_ w310]
              tunnel: w298 -> [_ w314]
              tunnel: [w304 w313] -> w297
              tunnel: w296 -> [_ w312]
              tunnel: w295 -> [w304 w306]
              frame False {
              }
              frame True {
                # "Clicks on the Symbol change state"
                n164 = property on="Property Node" class="Tree (strict)"(reference=w312, error in=w306, "Active Item Tag"=w310) -> (reference out=w311:refnum<vi>, error out=w305:errorcluster, "Glyph"=w309:i32)
                n165 = Equal?(x=37, y=w309) -> (x = y?=w307:bool)
                n166 = Build Array(w310) -> (w315:string[])
                n167 = call "SLSC-12201 Enable_Disable Channel.vi"("Item Ref in"=w314, "error in (no error)"=w305, "Enable"=w307, "Tree"=w315, "TreeControl in"=w311) -> ("error out"=w313:errorcluster)  [unwired: 5 in, 1 out]
              }
            }
          }
          event "Enable", "Disable": Value Change {
            n168 = event-data() -> ()  [unwired: 2 out]
            n169 = local read "Tree"() -> (w322:string[])
            n170 = control-ref of="Tree"() -> (w316:refnum<vi>)
            n171 = call "SLSC-12201 Enable_Disable Channel.vi"("Item Ref in"=w321, "error in (no error)"=w318, "Enable"="Enable", "Tree"=w322, "TreeControl in"=w316) -> ("error out"=w317:errorcluster, "Boolean"=w319:bool)  [unwired: 5 in]
            n172 = local write "Disable"(w319) -> ()
            n173 = local write "Enable"(w319) -> ()
          }
          event "Apply": Value Change {
            n174 = event-data() -> ()  [unwired: 2 out]
            n175 = property on="Direction" class="Ring (strict)"() -> ("Strings []"=w325:string[])  [unwired: 2 in, 2 out]
            n176 = local read "Tree"() -> (w333:string[])
            n177 = Index Array(array=w325, index="Direction") -> (element=w323:string)
            n178 = for {
              tunnel: w333 -> [w346] mode=indexing
              tunnel: w323 -> [w348]
              tunnel: w332 -> [w347]
              tunnel: "Direction" -> [w344]
              tunnel: [w342] -> w331
              tunnel: "/" ("regular expression") -> [w334]
              tunnel: "Line " ("string") -> [w339]
              tunnel: "Direction" ("Item Name") -> [w338]
              shift-right: [w335] -> w326
              shift-left: w327 -> [w337]
              n179 = Match Pattern(string=w346, regular expression=w334) -> (before substring=w341:string, after substring=w343:string)  [unwired: 1 in, 2 out]
              n180 = String Length(string=w343) -> (length=w352:i32)
              n181 = call-poly <vilib>:"NI VeriStand - Search for Item.vi"("error in"=w337, "Item Name"=w341, "Section Ref in"=w347) -> ("error out"=w336:errorcluster, "Item Ref"=w345:T2)  [unwired: 5 in, 2 out]
              n182 = Equal To 0?(x=w352) -> (x = 0?=w340:bool)
              n183 = Select(t=8, s=w340, f=1) -> (s? t:f=w351:i32)
              n184 = for {
                N: w351 -> [_]
                tunnel: w341 -> [w371]
                tunnel: w348 -> [w353]
                tunnel: w345 -> [w372]
                tunnel: w344 -> [w354]
                tunnel: w340 -> [w368]
                tunnel: w343 -> [w365]
                tunnel: [FALSE] -> w342
                tunnel: w339 -> [w363]
                tunnel: w338 -> [w362]
                shift-right: [w358] -> w335
                shift-left: w336 -> [w361]
                tunnel: w334 -> [w357]
                i -> [w374]
                n185 = Number To Decimal String(number=w374) -> (decimal integer string=w373:string)  [unwired: 1 in]
                n186 = Concatenate Strings(w363, w373) -> (w367:string)
                n187 = Select(t=w367, s=w368, f=w365) -> (s? t:f=w366:string)
                n188 = call-poly <vilib>:"NI VeriStand - Search for Item.vi"("error in"=w361, "Item Name"=w366, "Section Ref in"=w372) -> ("error out"=w360:errorcluster, "Item Ref"=w370:T2)  [unwired: 5 in, 2 out]
                n189 = Concatenate Strings(w371, w357, w366) -> (w356:string)
                n190 = call-poly <vilib>:"NI VeriStand - Search for Item.vi"("error in"=w360, "Item Name"=w362, "Section Ref in"=w370) -> ("error out"=w359:errorcluster, "Item Ref"=w369:T2)  [unwired: 5 in, 2 out]
                n191 = property on="Tree" class="Tree (strict)"("Active Item Tag"=w356, "ActiveColNum"=1 ("Active Cell:Active Column Number"), "Cell String"=w353) -> ()  [unwired: 2 in, 2 out]
                n192 = call <vilib>:"NI VeriStand - Set Custom Device Channel Default Value.vi"("error in (no error)"=w359, "Default Value"=w354, "Channel Ref in"=w369) -> ("error out"=w358:errorcluster)  [unwired: 7 in, 1 out]
              }
            }
            n193 = local write "Apply"(w331) -> ()
          }
          event "rev A": Value Change {
            n194 = event-data() -> ("NewVal"=w377:bool)  [unwired: 1 out]
            n195 = Not(x=w377) -> (.not. x?=w381:bool)
            n196 = call-poly <vilib>:"NI VeriStand - Set Item Property.vi"("error in (no error)"=w376, "Value"=w377, "Property Name"=w378, "Item Ref in"=w380) -> ("error out"=w375:errorcluster, "Item Ref out"=w379:T2)  [unwired: 5 in, 1 out]
            n197 = property on="Pullup Resistor Bank 0" class="Bool (strict)"("Visible"=w381) -> ()  [unwired: 2 in, 2 out]
            n198 = property on="Pullup Resistor Bank 1" class="Bool (strict)"("Visible"=w381) -> ()  [unwired: 2 in, 2 out]
            n199 = case shown="False" w377 {
              tunnel: w379 -> [w415 w463]
              tunnel: w375 -> [w411 w474]
              tunnel: [w395 w466] -> w382
              frame False {
                n200 = global read "Constants.vi" "Bank 0"() -> (w413:string)
                n201 = global read "Constants.vi" "Bank 1"() -> (w414:string)
                n202 = global read "Constants.vi" "SLSCChannelPath"() -> (w392:string)
                n203 = global read "Constants.vi" "GUID Channel Interface"() -> (w393:string)
                n204 = Build Array(w413, w414) -> (w412:string[])
                n205 = for {
                  tunnel: w412 -> [w455] mode=indexing
                  shift-right: [w443] -> w400
                  shift-left: w411 -> [w444]
                  tunnel: [w442] -> w410 mode=indexing
                  tunnel: w392 -> [w441]
                  tunnel: w393 -> [w440]
                  shift-right: [w438] -> w402
                  shift-left: w415 -> [w456]
                  i -> [w451]
                  n206 = call "SLSC Create Bank Properties.vi"("Bank Number"=w451) -> ("Outgoing configuration"=w450:T7[])  [unwired: 9 in, 1 out]
                  n207 = call-poly <vilib>:"NI VeriStand - Search for Item.vi"("error in"=w444, "Item Name"=w455, "Section Ref in"=w456) -> ("error out"=w445:errorcluster, "Item Ref"=w452:T2, "Section Ref out"=w438:T2)  [unwired: 5 in, 1 out]
                  n208 = Index Array(array=w450, index=4) -> (element=w448:T7)
                  n209 = Unbundle(w448) -> ("Channel Name"=w447:string, "SLSC Name"=w446:string, "Configuration"=w442:T4)  [unwired: 2 out]
                  n210 = call <vilib>:"NI VeriStand - Add Custom Device Channel.vi"("GUID (Default Channel)"=w440, "error in (no error)"=w445, "Channel"=w442, "Channel Name"=w447, "Parent Ref in"=w452) -> ("error out"=w453:errorcluster, "Channel Ref"=w454:T2)  [unwired: 3 in, 2 out]
                  n211 = call-poly <vilib>:"NI VeriStand - Set Item Property.vi"("Binary String (T)"=FALSE, "error in (no error)"=w453, "Value"=w446, "Property Name"=w441, "Item Ref in"=w454) -> ("error out"=w443:errorcluster)  [unwired: 4 in, 2 out]
                }
                n212 = Index Array(array=w410) -> (element #1=w409:T4, element #2=w408:T4)  [unwired: 2 in]
                n213 = Unbundle By Name(w409) -> ("Default Value"=w407:dbl)
                n214 = Unbundle By Name(w408) -> ("Default Value"=w405:dbl)
                n215 = Not Equal To 0?(x=w407) -> (x != 0?=w406:bool)
                n216 = Not Equal To 0?(x=w405) -> (x != 0?=w404:bool)
                n217 = local write "Pullup Resistor Bank 0"(w406) -> ()
                n218 = local write "Pullup Resistor Bank 1"(w404) -> ()
                n219 = global read "Constants.vi" "Command Channel"() -> (w391:string)
                n220 = call "SLSC Create Commands.vi"() -> ("Outgoing configuration"=w384:T11)  [unwired: 11 in]
                n221 = global read "Constants.vi" "Status Channel"() -> (w401:string)
                n222 = call "SLSC Create Status.vi"() -> ("Outgoing configuration"=w387:T11)  [unwired: 11 in]
                n223 = Array Subset(array=w384, index=3) -> (w383:T11)  [unwired: 1 in]
                n224 = call-poly <vilib>:"NI VeriStand - Search for Item.vi"("error in"=w400, "Item Name"=w401, "Section Ref in"=w402) -> ("error out"=w403:errorcluster, "Item Ref"=w399:T2, "Section Ref out"=w394:T2)  [unwired: 5 in, 1 out]
                n225 = Array Subset(array=w387, index=3) -> (w386:T11)  [unwired: 1 in]
                n226 = global read "Constants.vi" "SLSCChannelPath"() -> (w390:string)
                n227 = global read "Constants.vi" "GUID Channel Interface"() -> (w389:string)
                n228 = for {
                  tunnel: w399 -> [w433]
                  shift-right: [w427] -> w396
                  shift-left: w403 -> [w432]
                  tunnel: w392 -> [w435]
                  tunnel: w393 -> [w434]
                  tunnel: w386 -> [w431] mode=indexing
                  n229 = Unbundle(w431) -> ("Channel Name"=w430:string, "SLSC Name"=w428:string, "Channel"=w429:T4)
                  n230 = call <vilib>:"NI VeriStand - Add Custom Device Channel.vi"("GUID (Default Channel)"=w434, "error in (no error)"=w432, "Channel"=w429, "Channel Name"=w430, "Parent Ref in"=w433) -> ("error out"=w436:errorcluster, "Channel Ref"=w437:T2)  [unwired: 3 in, 2 out]
                  n231 = call-poly <vilib>:"NI VeriStand - Set Item Property.vi"("error in (no error)"=w436, "Value"=w428, "Property Name"=w435, "Item Ref in"=w437) -> ("error out"=w427:errorcluster)  [unwired: 5 in, 2 out]
                }
                n232 = call-poly <vilib>:"NI VeriStand - Search for Item.vi"("error in"=w396, "Item Name"=w391, "Section Ref in"=w394) -> ("error out"=w397:errorcluster, "Item Ref"=w398:T2)  [unwired: 5 in, 2 out]
                n233 = for {
                  tunnel: w398 -> [w421]
                  shift-right: [w424] -> w395
                  shift-left: w397 -> [w420]
                  tunnel: w390 -> [w423]
                  tunnel: w389 -> [w422]
                  tunnel: w383 -> [w419] mode=indexing
                  n234 = Unbundle(w419) -> ("Channel Name"=w418:string, "SLSC Name"=w416:string, "Channel"=w417:T4)
                  n235 = call <vilib>:"NI VeriStand - Add Custom Device Channel.vi"("GUID (Default Channel)"=w422, "error in (no error)"=w420, "Channel"=w417, "Channel Name"=w418, "Parent Ref in"=w421) -> ("error out"=w425:errorcluster, "Channel Ref"=w426:T2)  [unwired: 3 in, 2 out]
                  n236 = call-poly <vilib>:"NI VeriStand - Set Item Property.vi"("error in (no error)"=w425, "Value"=w416, "Property Name"=w423, "Item Ref in"=w426) -> ("error out"=w424:errorcluster)  [unwired: 5 in, 2 out]
                }
              }
              frame True {
                w467 = FALSE ("Pullup Resistor Bank 0")
                # "don't connect Rev A input"
                n237 = call "SLSC Create Bank Properties.vi"() -> ("Outgoing configuration"=w471:T7[])  [unwired: 10 in, 1 out]
                n238 = Index Array(array=w471, index=4) -> (element=w469:T7)
                n239 = Unbundle(w469) -> ("Channel Name"=w468:string)  [unwired: 4 out]
                n240 = call-poly <vilib>:"NI VeriStand - Search for Item.vi"("error in"=w474, "Item Name"=w468, "Section Ref in"=w463) -> ("error out"=w472:errorcluster, "Item Refs"=w473:T2[])  [unwired: 5 in, 2 out]
                n241 = call "SLSC Create Commands.vi"() -> ("Outgoing configuration"=w459:T11)  [unwired: 11 in]
                n242 = call "SLSC Create Status.vi"() -> ("Outgoing configuration"=w464:T11)  [unwired: 11 in]
                n243 = for {
                  tunnel: w473 -> [w489] mode=indexing
                  shift-right: [w487] -> w462
                  shift-left: w472 -> [w488]
                  n244 = call <vilib>:"NI VeriStand - Remove Custom Device Item.vi"("error in (no error)"=w488, "Force Delete (F)"=TRUE, "Item Ref in"=w489) -> ("error out"=w487:errorcluster)  [unwired: 7 in, 1 out]
                }
                n245 = Array Subset(array=w464, index=3) -> (w461:T11)  [unwired: 1 in]
                n246 = Array Subset(array=w459, index=3) -> (w457:T11)  [unwired: 1 in]
                n247 = Build Array (concatenate)(w461, w457) -> (w458:T11)
                n248 = for {
                  tunnel: w463 -> [w479]
                  shift-right: [w481] -> w466
                  shift-left: w462 -> [w478]
                  tunnel: w458 -> [w477] mode=indexing
                  n249 = Unbundle(w477) -> ("Channel Name"=w476:string)  [unwired: 2 out]
                  n250 = call-poly <vilib>:"NI VeriStand - Search for Item.vi"("error in"=w478, "Item Name"=w476, "Section Ref in"=w479) -> ("error out"=w480:errorcluster, "Item Refs"=w475:T2[])  [unwired: 5 in, 2 out]
                  n251 = for {
                    tunnel: w475 -> [w485] mode=indexing
                    shift-right: [w483] -> w481
                    shift-left: w480 -> [w484]
                    n252 = call <vilib>:"NI VeriStand - Remove Custom Device Item.vi"("error in (no error)"=w484, "Force Delete (F)"=TRUE, "Item Ref in"=w485) -> ("error out"=w483:errorcluster)  [unwired: 7 in, 1 out]
                  }
                }
                n253 = local write "Pullup Resistor Bank 0"(w467) -> ()
                n254 = local write "Pullup Resistor Bank 1"(w467) -> ()
              }
            }
          }
        }
        n255 = call <vilib>:"Simple Error Handler.vi"("error in (no error)"=w160) -> ("error out"=w159:errorcluster)  [unwired: 1 in, 7 out]
        n256 = call <vilib>:"Clear Errors.vi"("error in (no error)"=w159) -> ("error out"=w158:errorcluster)  [unwired: 1 in, 5 out]
      }
      n257 = Unregister For Events(event registration refnum=w152, error in=w151) -> (error out=w150:errorcluster)
    }
    frame Error {
      n258 = call <vilib>:"Simple Error Handler.vi"("error in (no error)"=w492) -> ("error out"=w491:errorcluster)  [unwired: 1 in, 7 out]
      n259 = call <vilib>:"Clear Errors.vi"("error in (no error)"=w491) -> ("error out"=w490:errorcluster)  [unwired: 1 in, 5 out]
    }
  }
  n260 = call <vilib>:"Clear Errors.vi"("error in (no error)"=w3) -> ()  [unwired: 5 in, 2 out]
  n261 = invoke class="VI" method="FP.Close"(error in=w26) -> (error out=w25:errorcluster)  [unwired: 2 in, 2 out]
  n262 = call <vilib>:"NI VeriStand - Signal When Ready for Shutdown.vi"("error in (no error)"=w25) -> ("error out"=→"error out":errorcluster)  [unwired: 10 out]
